vi "getNotifierServerStatus.vi"(8 "error in (no error)":errorcluster, 10 "notifier timeout":i32, 11 "TcpServerBase in":refnum<class "TcpServerBase.lvclass">) -> (0 "error out":errorcluster, 1 "timeout?":bool, 2 "connStatusCluster":T1, 3 "TcpServerBase out":refnum<class "TcpServerBase.lvclass">)   [LabVIEW 2018, in "TcpServerBase.lvclass"]
doc: "Get the notifierServerStatus from tcpServerStateMachine.vi.\n\nNote: Put this VI in Prealocated reentrant clone execution."
uses:
  TcpServerBase.lvclass
  TcpServerBase.lvclass/TcpServerBase.ctl
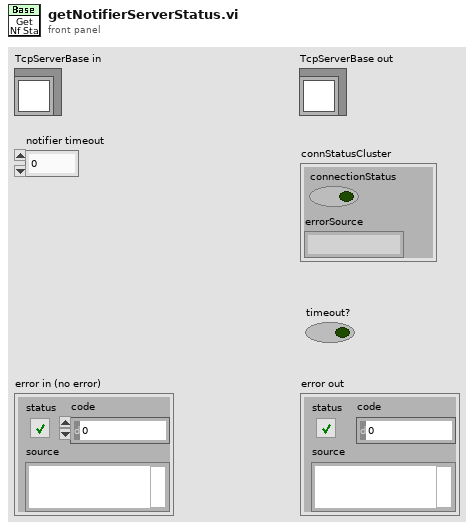
[diagram p1: front panel]
types:
  T1 = cluster{"connectionStatus":bool, "errorSource":string}
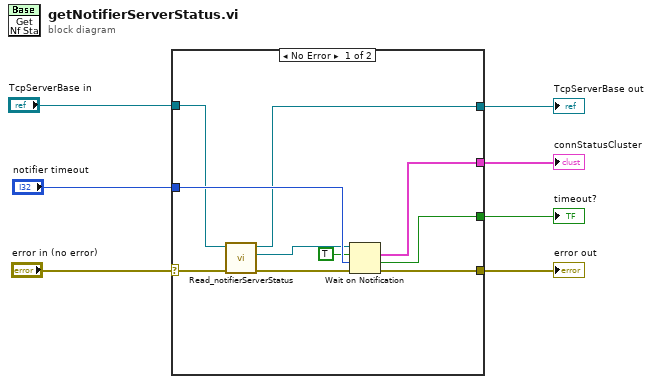
[diagram p0: block diagram]
diagram:
  n1 = case shown="No Error" "error in (no error)" {
    selector: "error in (no error)" -> [w16 w19]
    tunnel: "notifier timeout" -> [w17 _]
    tunnel: "TcpServerBase in" -> [w15 w18]
    tunnel: [w9 w19] -> w4
    tunnel: [w14 _] -> w3
    tunnel: [w11 _] -> w2
    tunnel: [w8 w18] -> w1
    frame No Error {
      n2 = call "Read_notifierServerStatus.vi"("error in (no error)"=w16, "TcpServerBase in"=w15) -> ("error out"=w10:errorcluster, "notifierServerStatus"=w13:refnum<notifier>, "TcpServerBase out"=w8:refnum<class "TcpServerBase.lvclass">)  [unwired: 7 in]
      n3 = Wait on Notification(notifier=w13, ignore previous (F)=TRUE, timeout in ms (-1)=w17, error in (no error)=w10) -> (notification=w14:T1, timed out?=w11:bool, error out=w9:errorcluster)  [unwired: 1 out]
    }
    frame Error {
    }
  }
  "error out" <- w4
  "connStatusCluster" <- w3
  "timeout?" <- w2
  "TcpServerBase out" <- w1
